vi "LVClass_HasoEngine Get Preferences.vi"(0 "HasoEngine in":refnum<class "HasoEngine.lvclass">, 11 "error in (no error)":errorcluster) -> (4 "HasoEngine out":refnum<class "HasoEngine.lvclass">, 6 "Slopes engine setup":T1={"Start sub-aperture"={"X"=0, "Y"=0}, "Pupil average"=670.0, "AutoStartSub-aperture"=FALSE} {"Pupil average" min=0.0 max=1.0}, 15 "error out":errorcluster)   [LabVIEW 2020, in "HasoEngine.lvclass"]
doc: "HasoSlopes computation preferences getter.\n\n--------------------------------------------------------------------------------\n\n<B>HasoEngineIn </B> : HasoEngine object.\n<B>HasoEngineOut </B> : HasoEngine object.\n<B>start_subpupil </B> : Coordinates of the first calculated sub-pupil (index coordinates relative to\n the top-left corner of the pupil).\n<B>denoising_strength </B> : Sensitivity of spot detection on summed images (between 0 and 1).\n<B>ErrorIn </B> : Error\n<B>ErrorOut </B> : Error\n\n--------------------------------------------------------------------------------"
uses:
  HasoEngine.lvclass
  SlopesEngineSetup.ctl
  Point2D.ctl
  HasoEngine.lvclass/HasoEngine.ctl
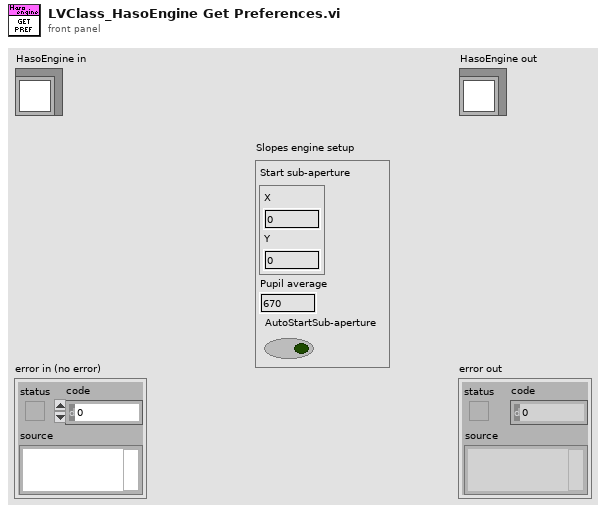
[diagram p1: front panel]
types:
  T1 = typedef "SlopesEngineSetup.ctl" = cluster{"Start sub-aperture":T2, "Pupil average":dbl, "AutoStartSub-aperture":bool}
  T2 = typedef "Point2D.ctl" = cluster{"X":u32, "Y":u32}
  T3 = typedef "ClassID.ctl" = i64
  T4 = cluster{"StartSubPupil":T2, "pupil_average":sgl, bool}
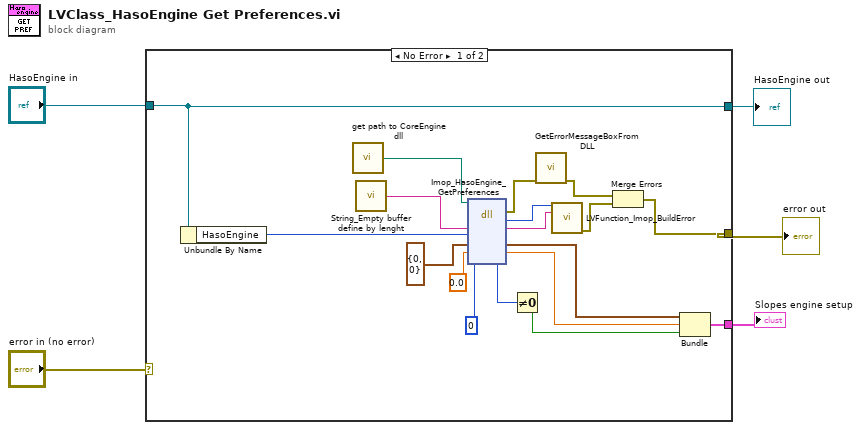
[diagram p0: block diagram]
diagram:
  n1 = case shown="No Error" "error in (no error)" {
    selector: "error in (no error)" -> [_ w24]
    tunnel: "HasoEngine in" -> [w13 w25]
    tunnel: [w13 w25] -> w2
    tunnel: [w9 w24] -> w3
    tunnel: [w14 _] -> w1
    frame No Error {
      n2 = Unbundle By Name(w13) -> ("HasoEngine"=w12:T3)
      n3 = call "get path to CoreEngine dll.vi"() -> ("path to wavekit library"=w20:path)  [unwired: 14 in, 1 out]
      n4 = call "String_Empty buffer define by lenght.vi"() -> ("Empty buffer"=w21:string)  [unwired: 1 in]
      n5 = dll-call lib="D:/2_trunk/Soft_haso/ImOpCoreEngine4_LV2011/DLLs/ImopEngine4_vc100.dll" fn="Imop_HasoEngine_GetPreferences"(path in=w20, "message"=w21, "objet"=w12, "StartSubPupil"=T2 {"X"=0, "Y"=0} ("dimension 2"), "pupil_average"=sgl 0.0, "AutoStartSub-aperture"=u8 0) -> (error out=w19:errorcluster, "return type"=w22:i32, "message"=w23:string, "StartSubPupil"=w16:T2, "pupil_average"=w15:sgl, "AutoStartSub-aperture"=w8:u8)  [unwired: 3 in, 1 out]
      n6 = Not Equal To 0?(x=w8) -> (x != 0?=w7:bool)
      n7 = call "GetErrorMessageBoxFromDLL.vi"("error IN"=w19) -> ("error OUT"=w11:errorcluster)  [unwired: 10 in]
      n8 = call "LVFunction_Imop_BuildError.vi"("code"=w22, "String to Prepend to source (\"\")"=w23) -> ("error out"=w10:errorcluster)  [unwired: 13 in]
      n9 = Merge Errors(w11, w10) -> (w9:errorcluster)
      n10 = Bundle("StartSubPupil"=w16, "pupil_average"=w15, w7) -> (w14:T4)  [unwired: 1 in]
    }
    frame Error {
    }
  }
  "error out" <- w3
  "HasoEngine out" <- w2
  "Slopes engine setup" <- w1
